vi "globals.vi"() -> ()   [LabVIEW 2013]
uses:
  qwtb_lvlib/TD Calculation Settings.ctl
  qwtb_lvlib/TD Uncertainty Calculation Method.ctl
  qwtb_lvlib/TD Correlation Calculation Settings.ctl
  qwtb_lvlib/TD DOF Calculation Settings.ctl
  qwtb_lvlib/TD MCM Calculation Settings.ctl
  qwtb_lvlib/TD MCM Calculation Method.ctl
  qwtb_lvlib/TD GUI Settings.ctl
  qwtb_lvlib/TD GUI Engine.ctl
  qwtb_lvlib/TD Algorithm Information.ctl
  qwtb_lvlib/TD Quantity.ctl
panel:
  out "Data Out Q list reference":refnum<vi>
  in  "Current Algorithm":T1
  in  "Data Out":T2[](array[typedef])
  in  "Data In":T2[](array[typedef])
  out "Available Algorithms":T1[](array[typedef])
  in  "GUI Settings":T3
  in  "Calculation Settings":T5={"Verbose"=FALSE, "Uncertainty Calculation Method"=enum."none", "Correlations"={"Required"=FALSE, "Generate"=TRUE}, "Degrees of Freedom"={"Required"=FALSE, "Generate"=TRUE}, "MCM Calculation Settings"={"Repeats"=100, "Verbose"=TRUE, "Parallelization method"=enum."Single Core", "Processors"=1, "Temporary directory"=".", "Randomize"=TRUE}} {"MCM Calculation Settings"."Processors" min=1 step=1; "MCM Calculation Settings"."Repeats" min=1 step=1}
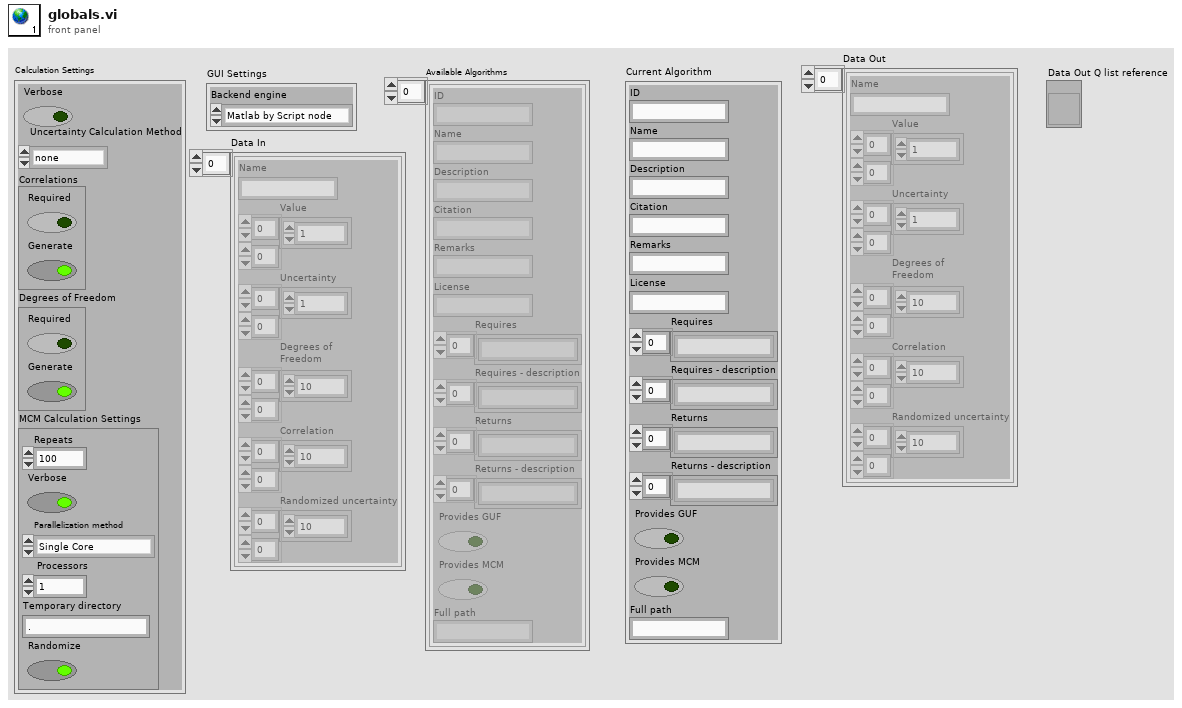
[diagram p1: front panel]
types:
  T1 = typedef "TD Algorithm Information.ctl" = cluster{"ID":string, "Name":string, "Description":string, "Citation":string, "Remarks":string, "License":string, "Requires":string[], "Requires - description":string[], "Returns":string[], "Returns - description":string[], "Provides GUF":bool, "Provides MCM":bool, "Full path":string}
  T2 = typedef "TD Quantity.ctl" = cluster{"Name":string, "Value":dbl[][], "Uncertainty":dbl[][], "Degrees of\nFreedom":dbl[][], "Correlation":dbl[][], "Randomized uncertainty":dbl[][]}
  T3 = typedef "TD GUI Settings.ctl" = cluster{"Backend engine":T4}
  T4 = typedef "TD GUI Engine.ctl" = enum16{"Matlab by Script node", "GNU Octave by GOLPI"}
  T5 = typedef "TD Calculation Settings.ctl" = cluster{"Verbose":bool, "Uncertainty Calculation Method":T6, "Correlations":T7, "Degrees of Freedom":T8, "MCM Calculation Settings":T9}
  T6 = typedef "TD Uncertainty Calculation Method.ctl" = enum16{"none", "GUF", "MCM"}
  T7 = typedef "TD Correlation Calculation Settings.ctl" = cluster{"Required":bool, "Generate":bool}
  T8 = typedef "TD DOF Calculation Settings.ctl" = cluster{"Required":bool, "Generate":bool}
  T9 = typedef "TD MCM Calculation Settings.ctl" = cluster{"Repeats":i32, "Verbose":bool, "Parallelization method":T10, "Processors":i32, "Temporary directory":string, "Randomize":bool}
  T10 = typedef "TD MCM Calculation Method.ctl" = enum16{"Single Core", "Multi Core", "Multi Station"}
diagram:
